vi "link_test_9024.vi"() -> ()   [LabVIEW 2019]
uses:
  RT Controls/MainBox Idle.ctl
  RT Controls/TopBox Json Reply.ctl
  RT Controls/TopBox Reply.ctl
  RT Controls/Top Dome Control.ctl
  RT Controls/Top Dome Status String.ctl
  RT Controls/TopBox Config.ctl
  <vilib>/Utility/error.llb/DialogType.ctl
panel:
  out "connect error":errorcluster
  out "topbox":T1 {"value"."DomeStatus"."LowerDoorEl" format="%.2f"; "value"."DomeStatus"."UpperDoorEl" format="%.2f"}
  out "json error":errorcluster
  out "error out":errorcluster
  in  "value":T6
  in  "stop":bool
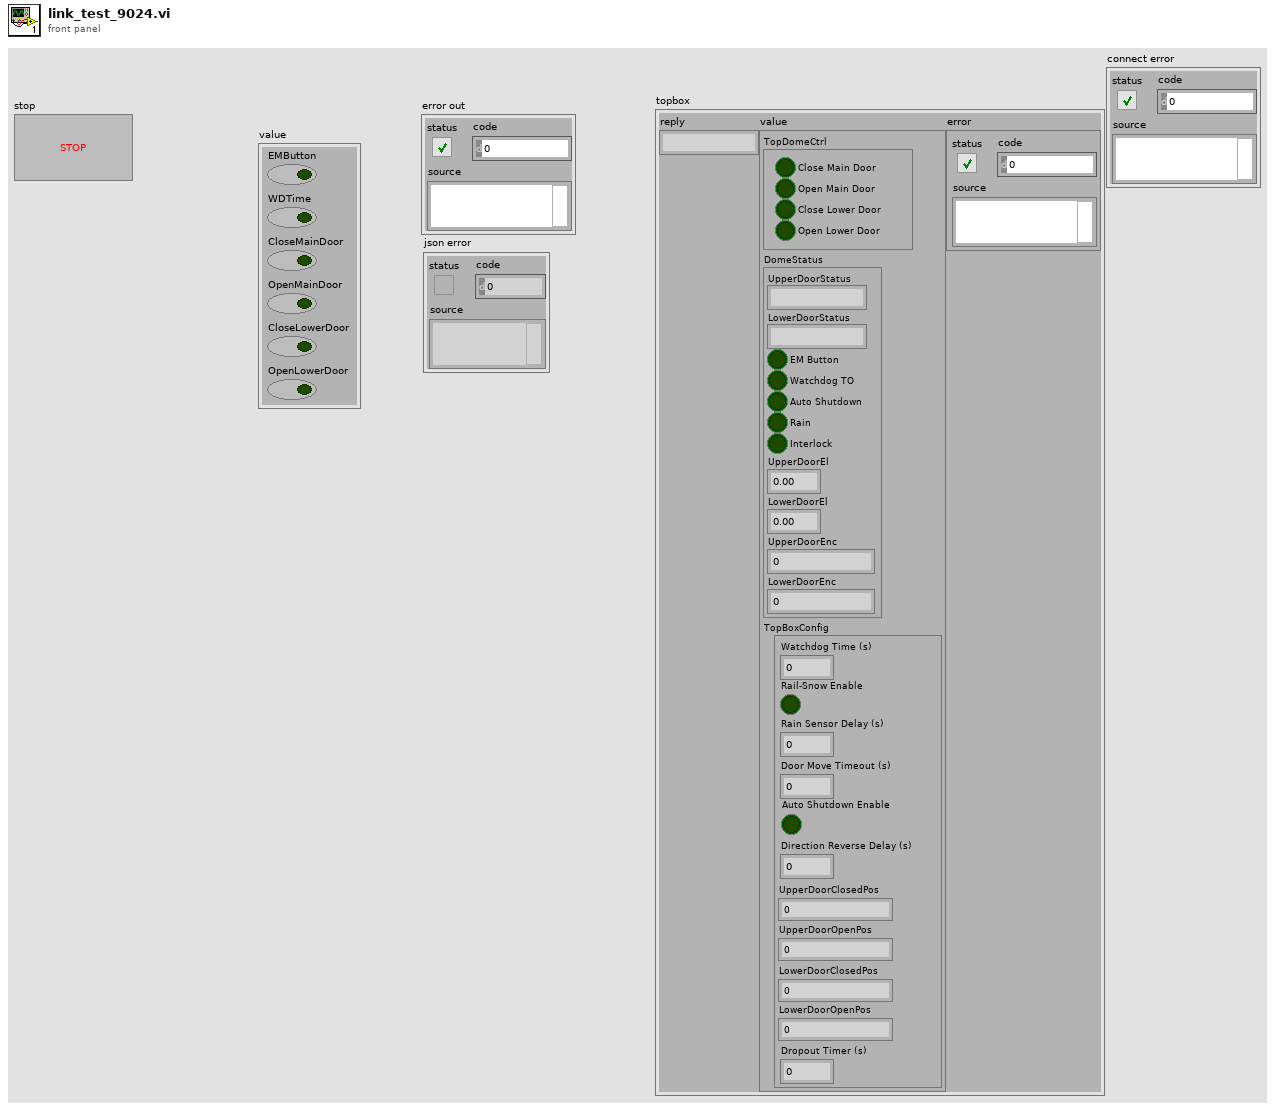
[diagram p1: front panel]
types:
  T1 = typedef "TopBox Json Reply.ctl" = cluster{"reply":string, "value":T2, "error":errorcluster}
  T2 = typedef "TopBox Reply.ctl" = cluster{"TopDomeCtrl":T3, "DomeStatus":T4, "TopBoxConfig":T5}
  T3 = typedef "Top Dome Control.ctl" = cluster{"OpenLowerDoor":bool, "CloseLowerDoor":bool, "OpenMainDoor":bool, "CloseMainDoor":bool}
  T4 = typedef "Top Dome Status String.ctl" = cluster{"UpperDoorStatus":string, "LowerDoorStatus":string, "EM Button":bool, "WDTime":bool, "AutoShut":bool, "Rain":bool, "Interlock":bool, "UpperDoorEl":dbl, "LowerDoorEl":dbl, "UpperDoorEnc":u64, "LowerDoorEnc":u64}
  T5 = typedef "TopBox Config.ctl" = cluster{"WatchdogTim":i32, "RainEn":bool, "DoorMoveTO":i32, "AutoShutEn":bool, "DirRevDel":i32, "UpperClosedEnc":u64, "UpperOpenEnc":u64, "LowerClosedEnc":u64, "LowerOpenEnc":u64, "RainTim":i32, "DropoutTim":i32}
  T6 = typedef "MainBox Idle.ctl" = cluster{"EMButton":bool, "WDTime":bool, "CloseMainDoor":bool, "OpenMainDoor":bool, "CloseLowerDoor":bool, "OpenLowerDoor":bool}
  T7 = typedef "DialogType.ctl" = u16
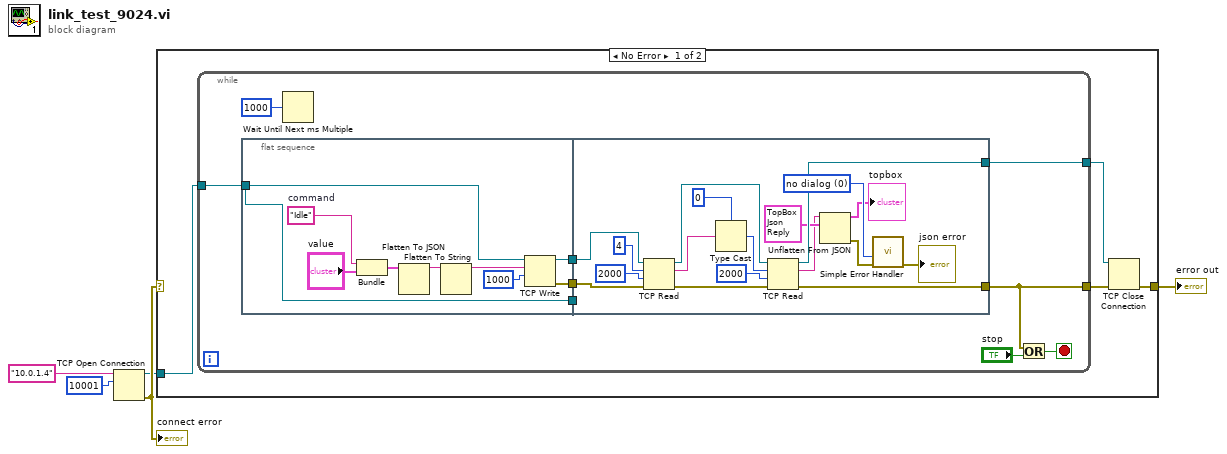
[diagram p0: block diagram]
diagram:
  n1 = TCP Open Connection(address="10.0.1.4", remote port or service name=u16 10001) -> (connection ID=w2:refnum<k5>, error out=w3:errorcluster)  [unwired: 3 in]
  "connect error" <- w3
  n2 = case shown="No Error" w3 {
    selector: w3 -> [_ w46]
    tunnel: w2 -> [w9 _]
    tunnel: [w6 w46] -> w1
    frame No Error {
      n3 = while {
        tunnel: w9 -> [w18]
        tunnel: [w17] -> w8
        tunnel: [w12] -> w7
        stop <- w11 stop-if-true
        n4 = flat-sequence {
          tunnel: w18 -> [w27]
          tunnel: [w27] -> w16
          tunnel: [w20] -> w15
          tunnel: [w19] -> w14
          tunnel: [w37] -> w17
          tunnel: [w36] -> w12
          tunnel: w16 -> [_]
          tunnel: w15 -> [w29]
          tunnel: w14 -> [w28]
          frame #0 {
            w21 = "Idle"  # command
            n5 = Bundle("command"=w21, "value"="value") -> (w23:cluster{"command":string, "value":T6})  [unwired: 1 in]
            n6 = Flatten To JSON(anything=w23) -> (JSON string=w24:string)  [unwired: 2 in, 1 out]
            n7 = Flatten To String(anything=w24) -> (data string=w25:string)  [unwired: 3 in, 2 out]
            n8 = TCP Write(connection ID=w27, data in=w25, 9:1000 ("timeout ms (25000)")) -> (connection ID out=w19:refnum<k5>, error out=w20:errorcluster)  [unwired: 1 in, 1 out]
          }
          frame #1 {
            w35 = T7 0 items=["no dialog", "OK message", "continue or stop message", "OK message + warnings", "continue/stop + warnings"] ("type of dialog (OK msg:1)")
            n9 = TCP Read(connection ID=w28, bytes to read=4, error in (no error)=w29, 9:2000 ("timeout ms (25000)")) -> (connection ID out=w43:refnum<k5>, data out=w44:string, error out=w42:errorcluster)  [unwired: 1 in]
            n10 = Type Cast(type=0 ("length"), x=w44) -> (*(type *) &x=w45:i32)
            n11 = TCP Read(connection ID=w43, bytes to read=w45, error in (no error)=w42, 9:2000 ("timeout ms (25000)")) -> (connection ID out=w37:refnum<k5>, data out=w32:string, error out=w36:errorcluster)  [unwired: 1 in]
            n12 = Unflatten From JSON(JSON string=w32, type and defaults=T1 {"reply"="", "value"={"TopDomeCtrl"={"OpenLowerDoor"=FALSE, "CloseLowerDoor"=FALSE, "OpenMainDoor"=FALSE, "CloseMainDoor"=FALSE}, "DomeStatus"={"UpperDoorStatus"="", "LowerDoorStatus"="", "EM Button"=FALSE, "WDTime"=FALSE, "AutoShut"=FALSE, "Rain"=FALSE, "Interlock"=FALSE, "UpperDoorEl"=0.0, "LowerDoorEl"=0.0, "UpperDoorEnc"=0, "LowerDoorEnc"=0}, "TopBoxConfig"={"WatchdogTim"=0, "RainEn"=FALSE, "DoorMoveTO"=0, "AutoShutEn"=FALSE, "DirRevDel"=0, "UpperClosedEnc"=0, "UpperOpenEnc"=0, "LowerClosedEnc"=0, "LowerOpenEnc"=0, "RainTim"=0, "DropoutTim"=0}}, "error"={"status"=FALSE, "code"=0, "source"=""}}) -> (value=→"topbox":T1, error out=w34:errorcluster)  [unwired: 5 in]
            n13 = call <vilib>:"Simple Error Handler.vi"("type of dialog (OK msg:1)"=w35, "error in (no error)"=w34) -> ("error out"=→"json error":errorcluster)  [unwired: 3 in, 4 out]
          }
        }
        n14 = Wait Until Next ms Multiple(millisecond multiple=u32 1000) -> ()  [unwired: 1 out]
        n15 = Or(x=w12, y="stop") -> (x .or. y?=w11:bool)
      }
      n16 = TCP Close Connection(connection ID=w8, error in (no error)=w7) -> (error out=w6:errorcluster)  [unwired: 1 in, 1 out]
    }
    frame Error {
    }
  }
  "error out" <- w1
